vi "Launcher.vi"() -> ()   [LabVIEW 2024]
uses:
  <vilib>/Utility/miscctls.llb/LVRectTypeDef.ctl
  Client/Client_class/Client.lvclass
  5928e640-d91e-4c91-af01-912b1cffb1fd.vi
panel:
  out "Cover Files":path[](array[path])
  in  "Stop":bool
  in  "Hamburger Menu Background":T1
  out "Current Song Name":string
  in  "Stop Button":bool
  in  "Skip Button":bool
  in  "PlayPause Button":bool
  in  "Rewind Button":bool
  out "Music Duration Slider":dbl(slide) scale=0.0..4.590585034013605
  out "Middle Pic":picture
  out "Left Pic":picture
  out "Right Pic":picture
  out "Left Pic 2":picture
  out "Right Pic 2":picture
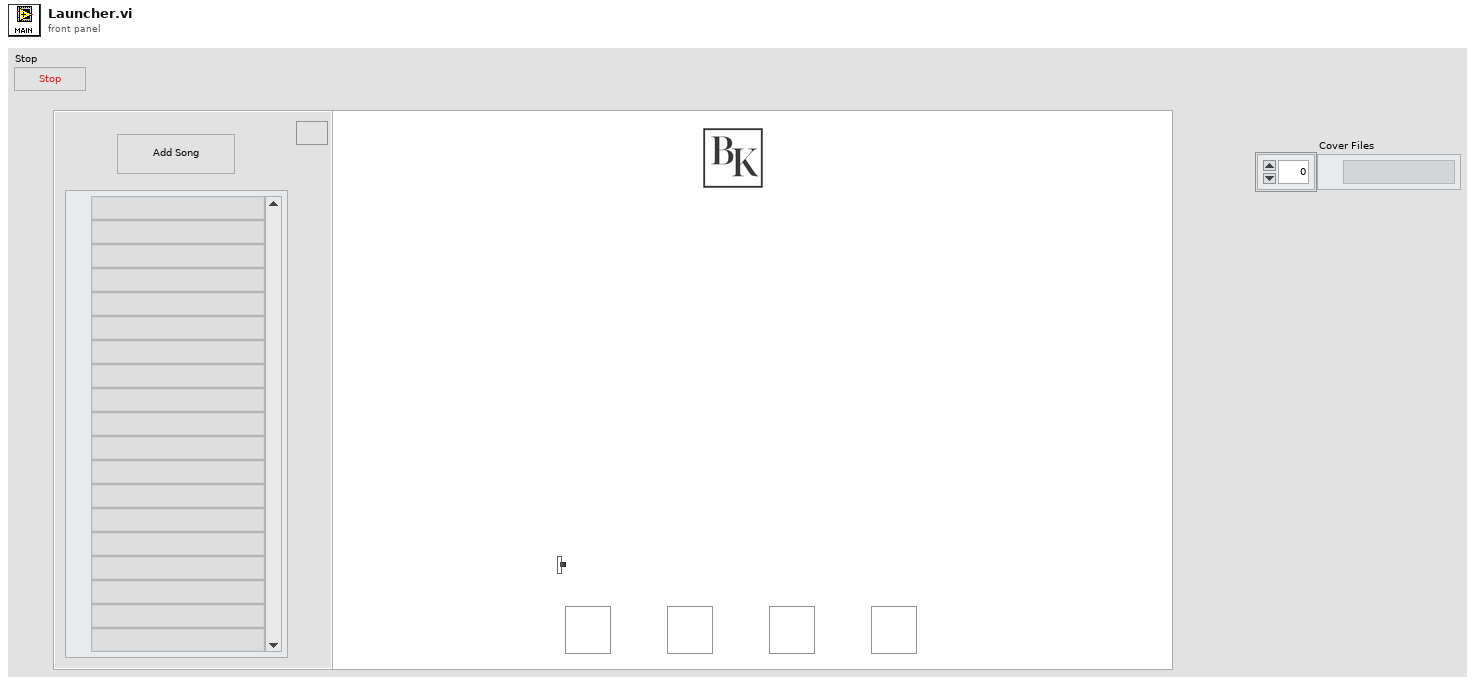
[diagram p1: front panel]
types:
  T1 = cluster{"Hamburger Menu":bool, "New Song":bool, "Song List":path[]}
  T2 = typedef "LVRectTypeDef.ctl" = cluster{"Left":i16, "Top":i16, "Right":i16, "Bottom":i16}
  T3 = cluster{"left":i16, "top":i16, "right":i16, "bottom":i16}
  T4 = typedef "MediaPlayer.lvclass/Current Info.ctl" = cluster{"Duration":dbl, "Name":string, "Is playing?":bool, "Current Music Index":i64}
  T5 = typedef "imagedata.ctl" = cluster{"image type":i32, "image depth":i32, "image":u8[], "mask":u8[], "colors":u32[], "Rectangle":cluster{"left":i16, "top":i16, "right":i16, "bottom":i16}}
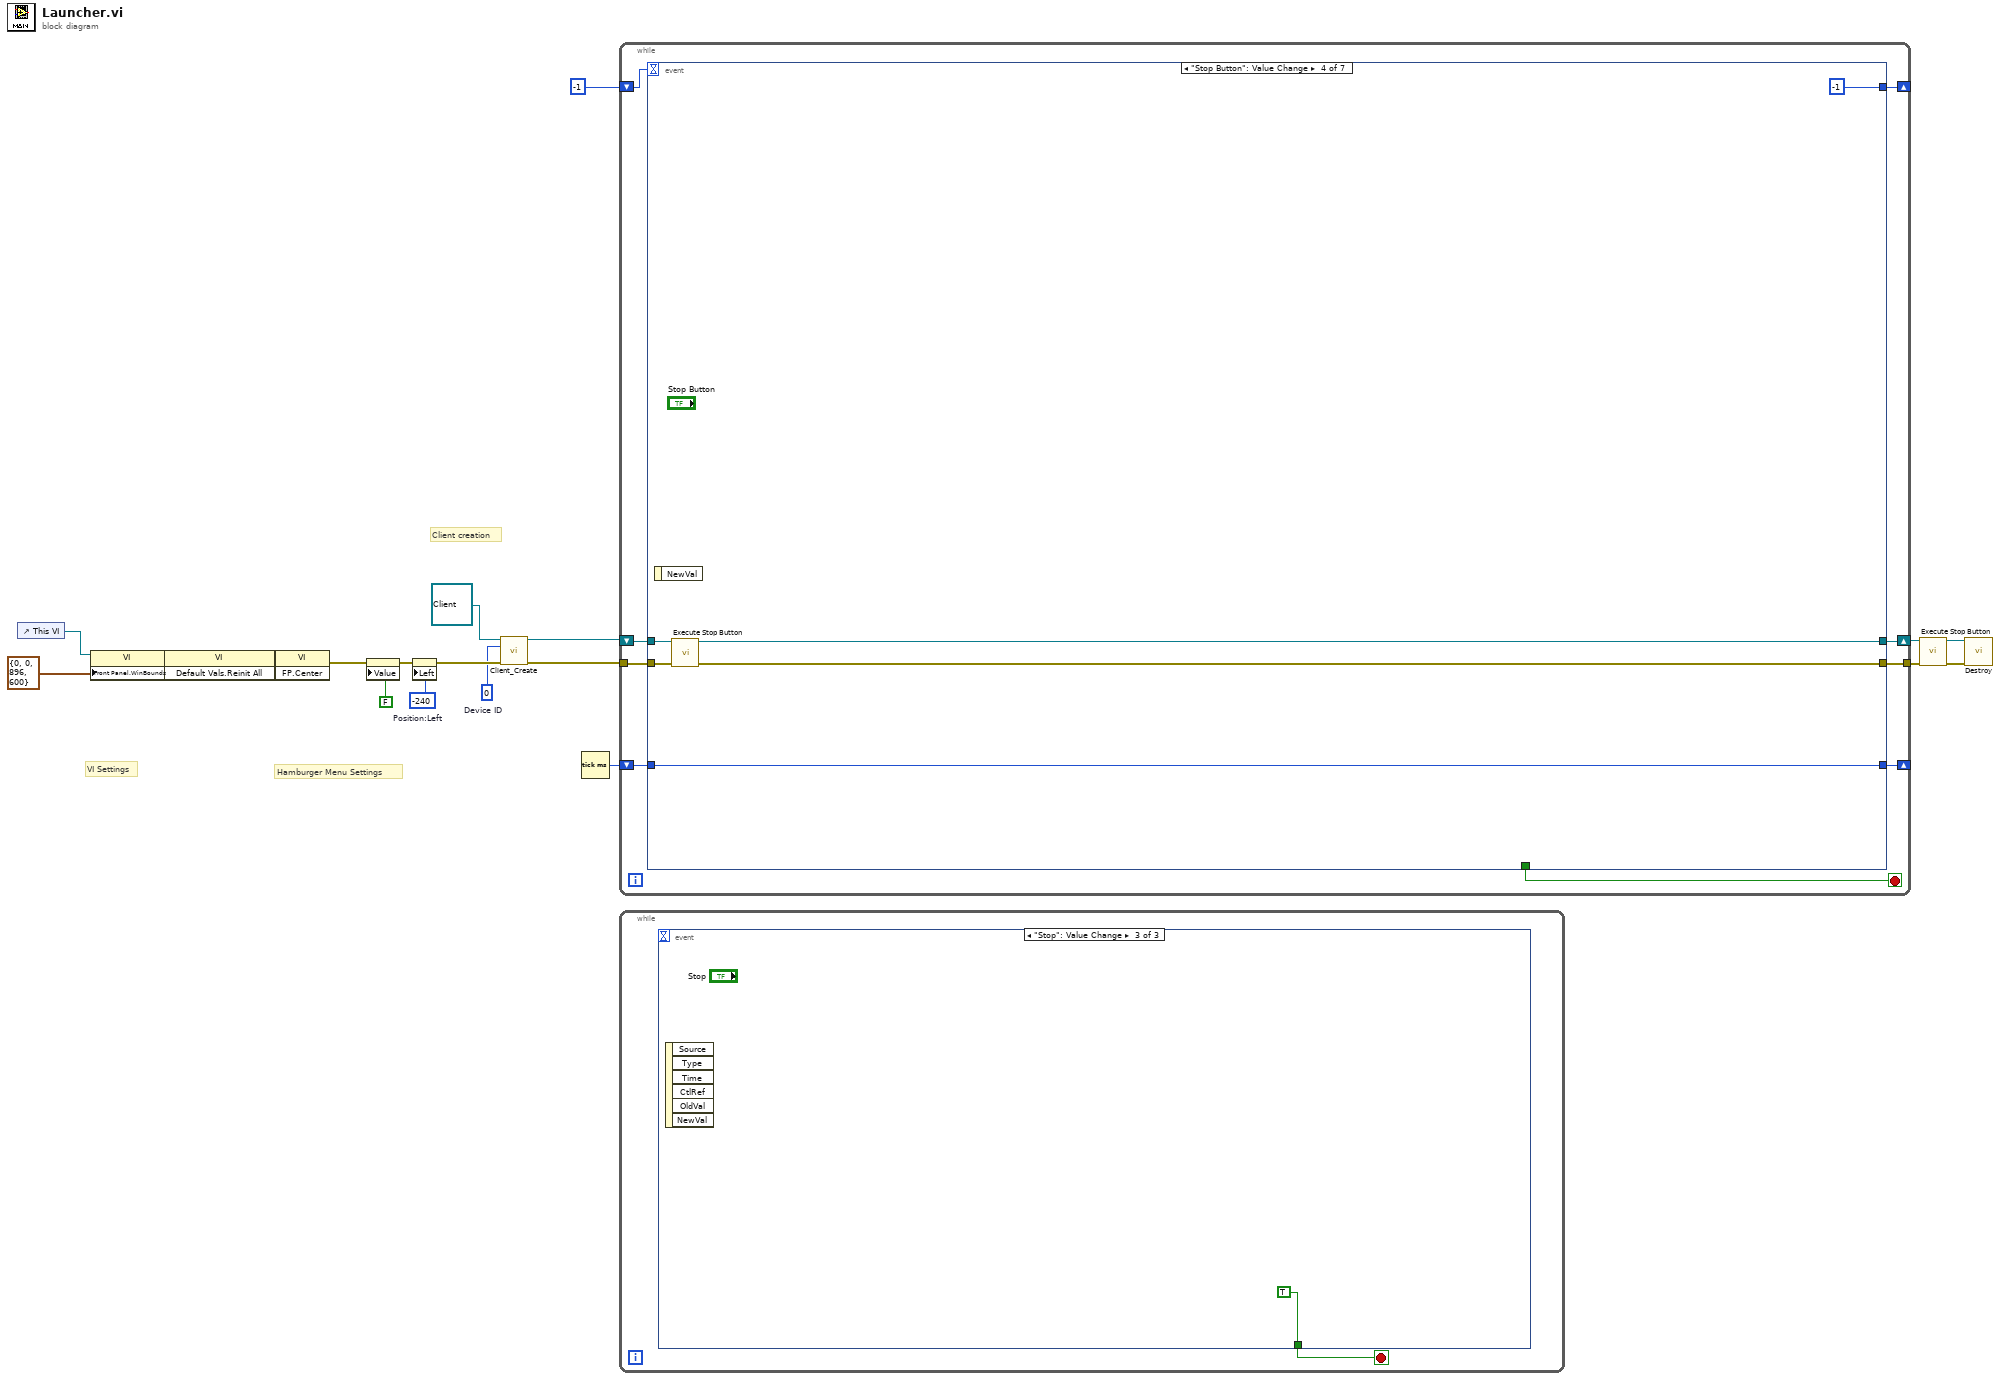
[diagram p0: block diagram]
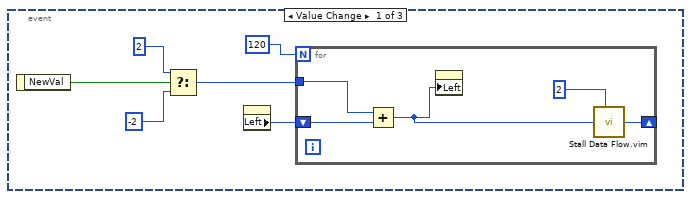
[diagram p2: hidden frame]
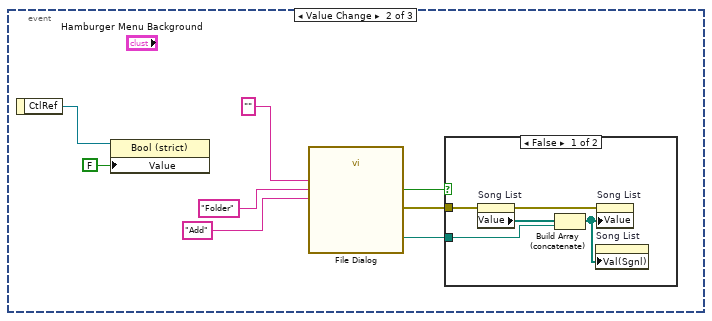
[diagram p3: hidden frame]
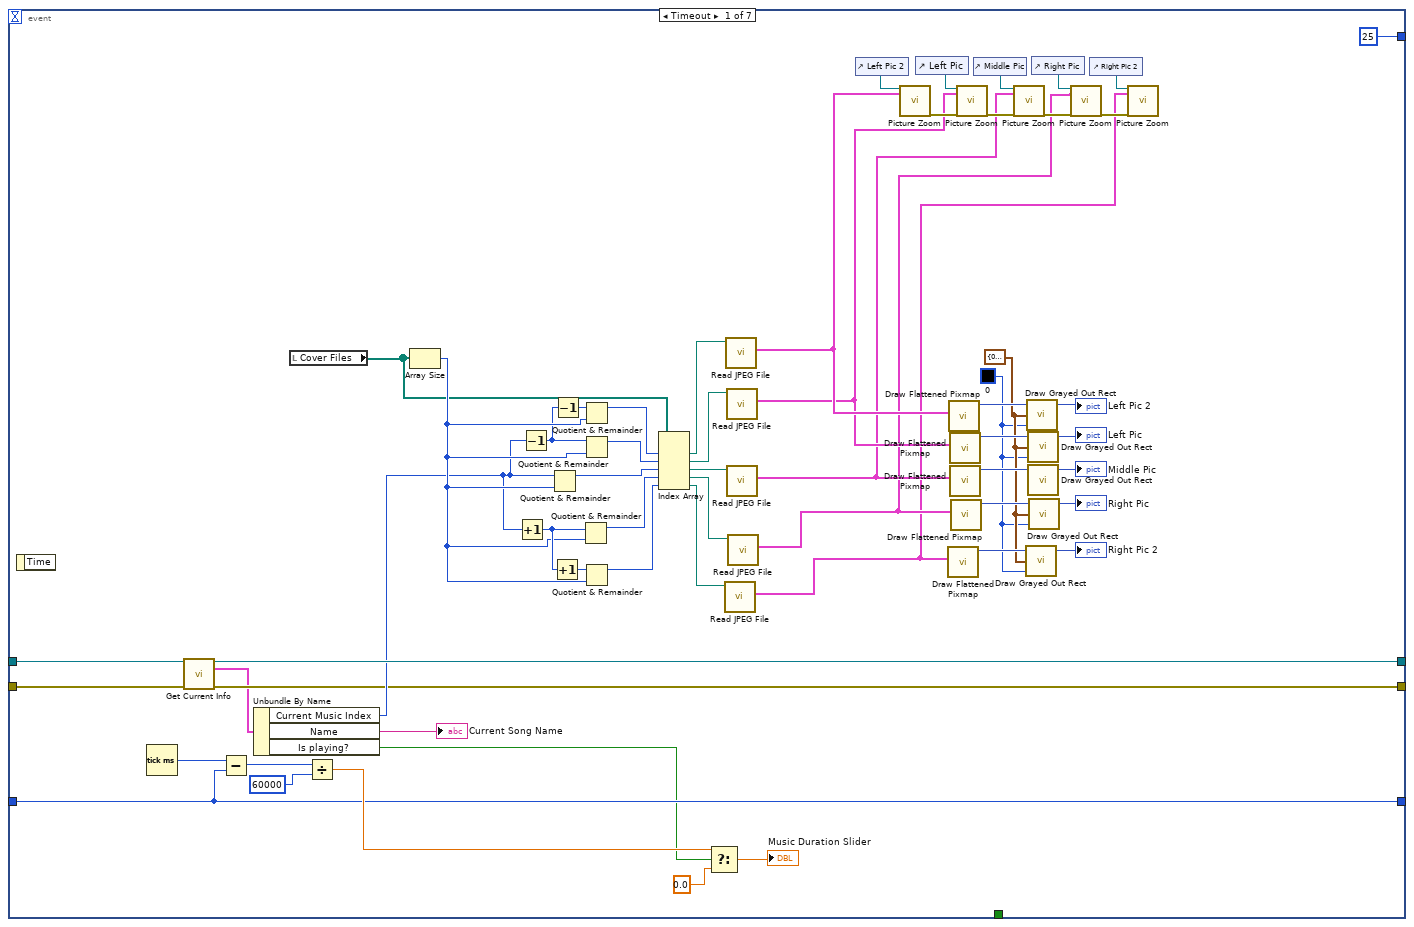
[diagram p5: hidden frame]
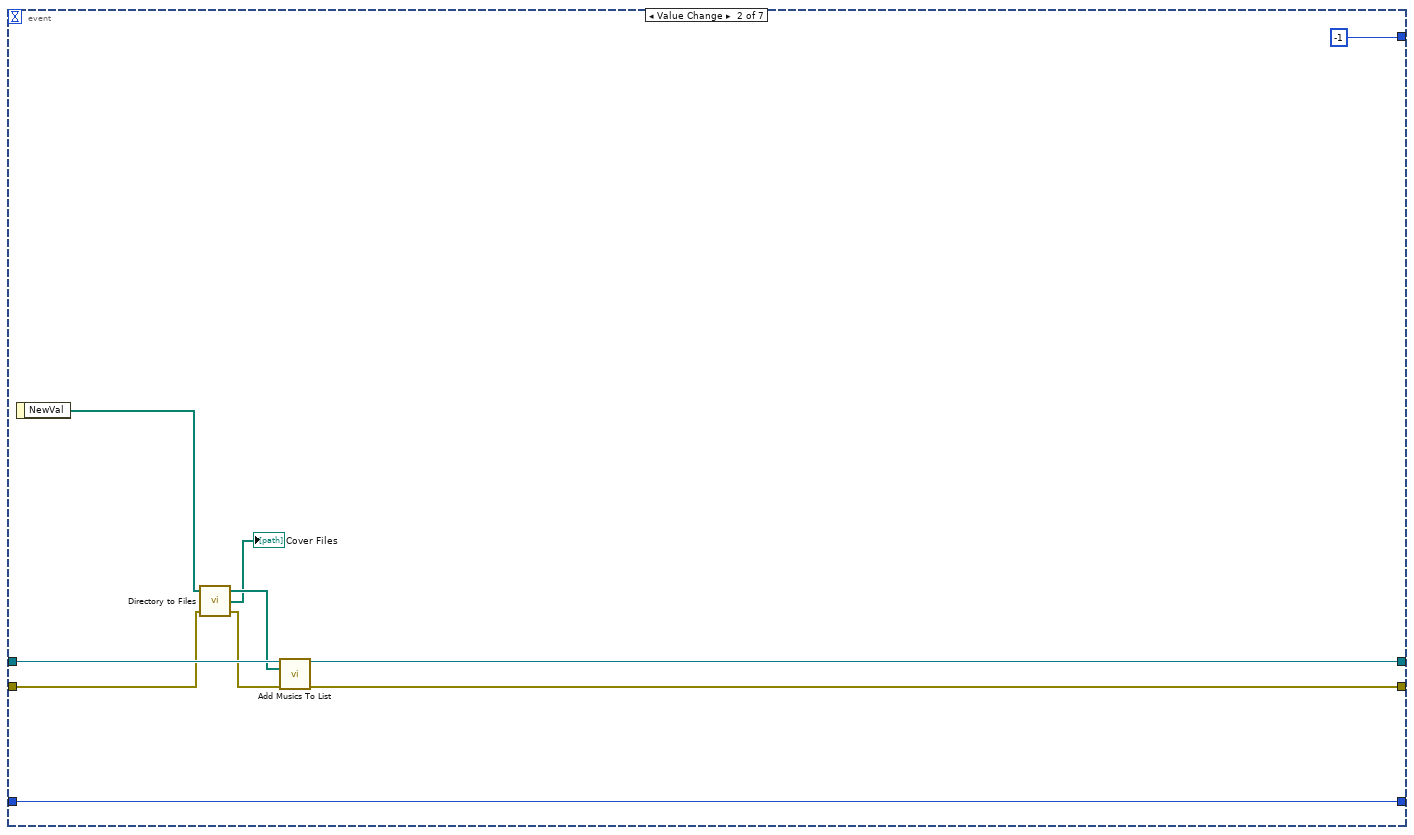
[diagram p6: hidden frame]
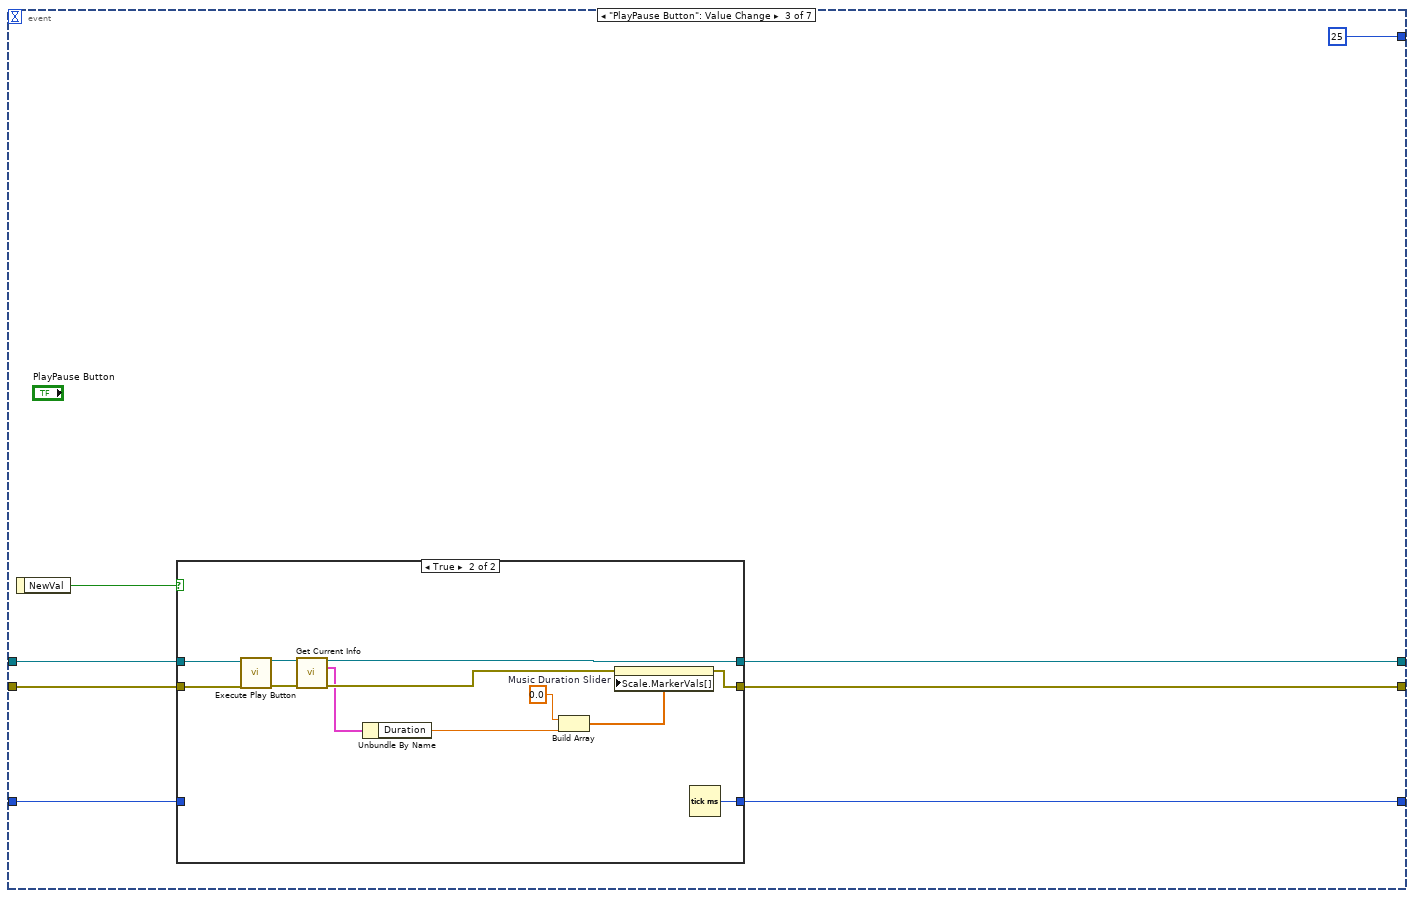
[diagram p7: hidden frame]
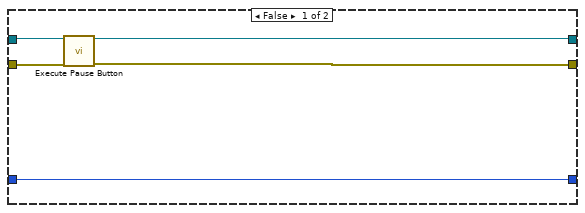
[diagram p8: hidden frame]
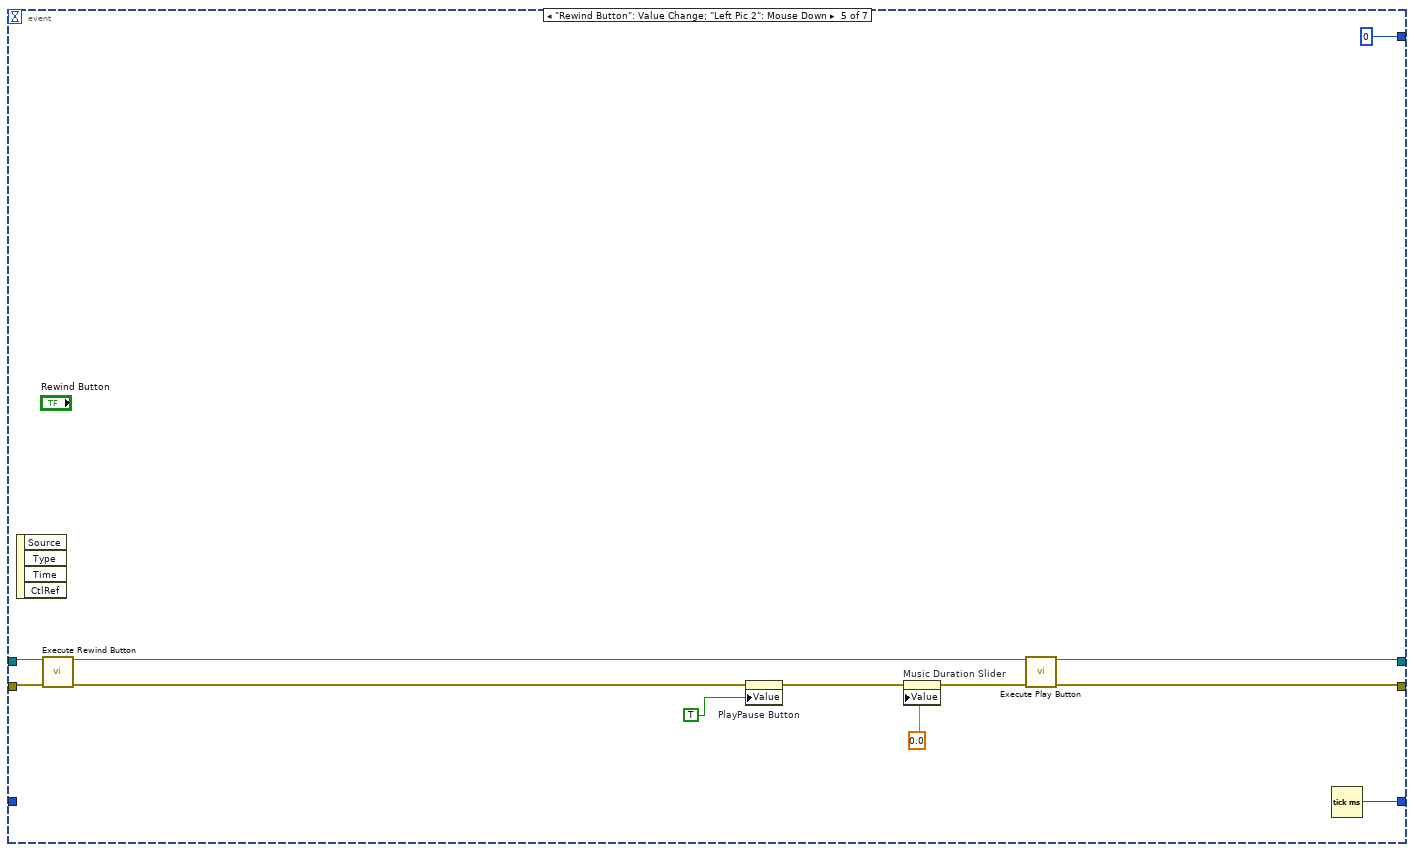
[diagram p9: hidden frame]
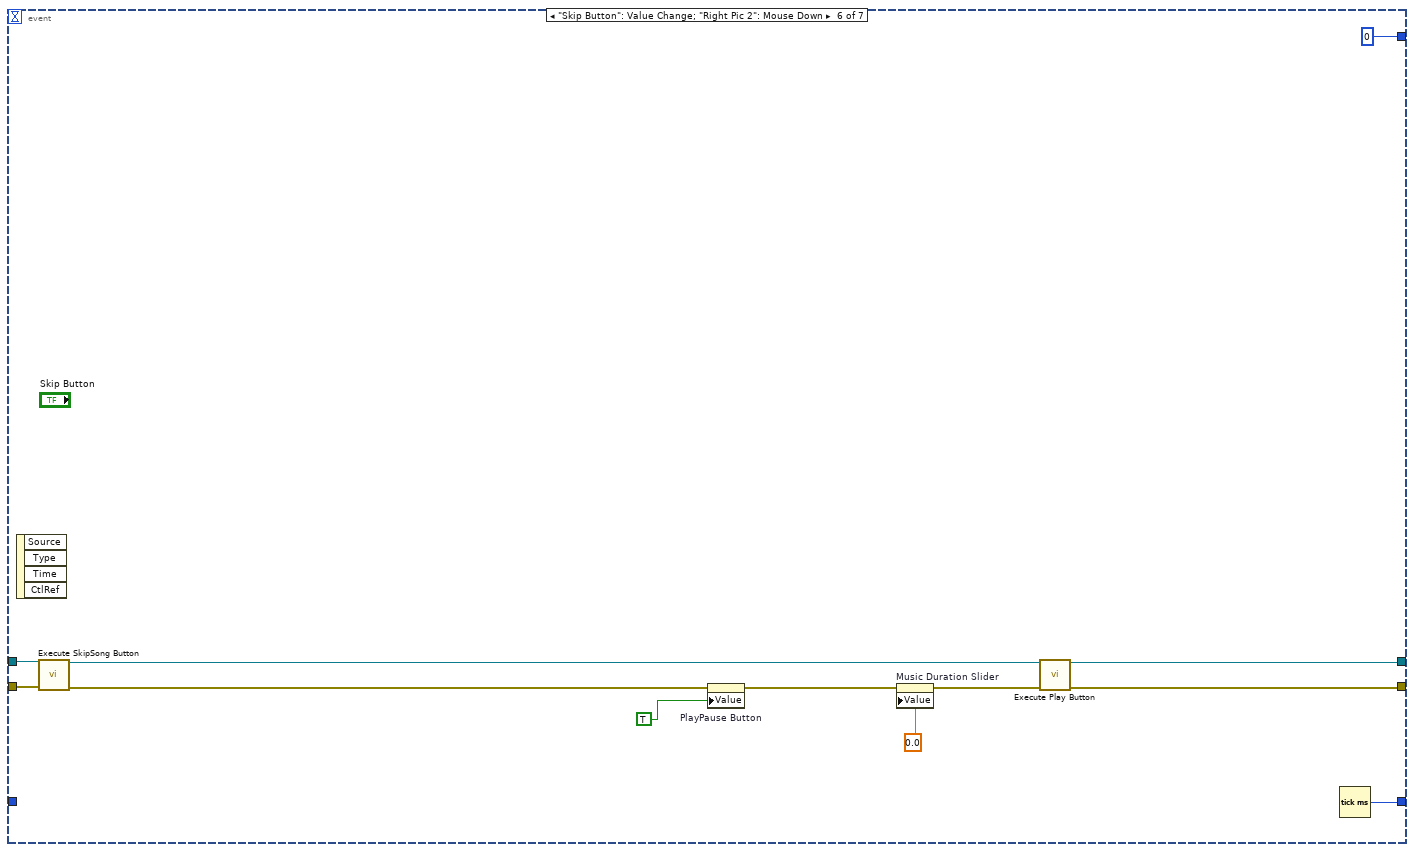
[diagram p10: hidden frame]
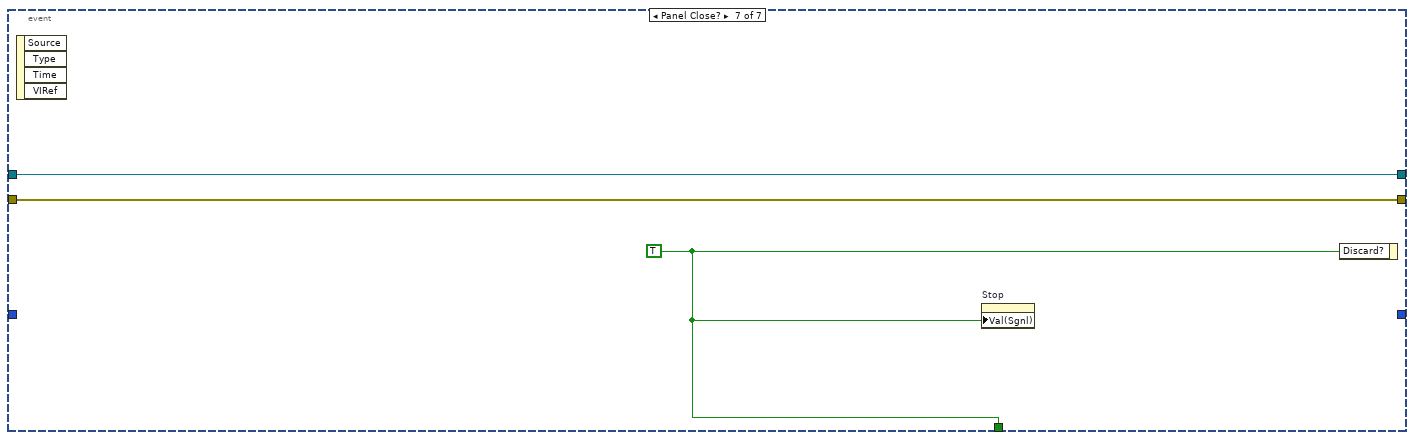
[diagram p11: hidden frame]
diagram:
  w3 = u32 0  # Device ID
  w18 = -240  # Position:Left
  # "Client creation"
  # "VI Settings"
  # "Hamburger Menu Settings"
  n1 = control-ref of="This VI"() -> (w20:refnum<vi>)
  n2 = property class="VI"(reference=w20, "Front Panel.WinBounds"=T2 {"Left"=0, "Top"=0, "Right"=896, "Bottom"=600} ("Front Panel Window:Window Bounds")) -> (reference out=w6:refnum<vi>, error out=w19:errorcluster)  [unwired: 1 in]
  n3 = invoke class="VI" method="Default Vals.Reinit All"(reference=w6, error in=w19) -> (reference out=w5:refnum<vi>, error out=w7:errorcluster)  [unwired: 1 in, 1 out]
  n4 = invoke class="VI" method="FP.Center"(reference=w5, error in=w7) -> (error out=w15:errorcluster)  [unwired: 1 in, 2 out]
  n5 = property on="Hamburger Menu" class="Bool (strict)"(error in=w15, "Value"=FALSE) -> (error out=w17:errorcluster)  [unwired: 1 in, 1 out]
  n6 = property on="Hamburger Menu Background" class="Clust (strict)"(error in=w17, "Left"=w18) -> (error out=w14:errorcluster)  [unwired: 1 in, 1 out]
  n7 = call "Client_Create.vi"("reference in"=refnum<class "Client.lvclass"> refnum ("Client"), "Device ID"=w3, "Error In"=w14) -> ("reference out"=w2:refnum<class "Client.lvclass">, "Error Out"=w1:errorcluster)  [unwired: 11 in]
  n8 = Tick Count (ms)() -> (millisecond timer value=w13:u32)
  n9 = while {
    shift-right: [w27] -> w9
    shift-left: w2 -> [w29]
    tunnel: w1 -> [w28]
    tunnel: [w26] -> w10
    shift-right: [w24] -> _
    shift-left: w13 -> [w25]
    shift-right: [w22] -> _
    shift-left: -1 -> [w23]
    stop <- w30 stop-if-true
    n10 = event shown="[3] \"Stop Button\": Value Change" {
      selector: _ -> [_ _ _ _ _ _ _]
      dyn-events: _ -> [_ _ _ _ _ _ _]
      timeout: w23 -> [_ _ _ _ _ _ _]
      tunnel: [_ _ _ _ _ _ w154] -> w30
      tunnel: w29 -> [w83 w95 w105 w128 w141 w152 w156]
      tunnel: w28 -> [w82 w92 w106 w129 w140 w153 w155]
      tunnel: [w84 w94 w103 w127 w136 w148 w156] -> w27
      tunnel: [w32 w96 w104 w126 w138 w150 w155] -> w26
      tunnel: w25 -> [w81 w97 w100 w125 _ _ _]
      tunnel: [w81 w97 w102 w125 w130 w142 _] -> w24
      tunnel: [25 -1 25 -1 0 0 _] -> w22
      event Timeout {
        w47 = u32 0 ("color(black)")
        w48 = T3 {"left"=0, "top"=0, "right"=1000, "bottom"=1000} ("rect")
        n11 = event-data() -> ()  [unwired: 1 in, 1 out]
        n12 = Tick Count (ms)() -> (millisecond timer value=w88:u32)
        n13 = call-dynamic "Get Current Info.vi"("reference in"=w83, "Error In"=w82) -> ("reference out"=w84:refnum<class "Client.lvclass">, "Current Info"=w31:T4, "Error Out"=w32:errorcluster)  [unwired: 11 in]
        n14 = Subtract(x=w88, y=w81) -> (x-y=w87:u32)
        n15 = Unbundle By Name(w31) -> ("Current Music Index"=w52:i64, "Name"=→"Current Song Name":string, "Is playing?"=w50:bool)
        n16 = local read "Cover Files"() -> (w67:path[])
        n17 = Divide(x=w87, y=u32 60000) -> (x/y=w85:dbl)
        n18 = Array Size(array=w67) -> (size(s)=w71:i32)
        n19 = Increment(x=w52) -> (x+1=w73:i64)
        n20 = Decrement(x=w52) -> (x-1=w70:i64)
        n21 = Quotient & Remainder(x=w52, y=w71) -> (x-y*floor(x/y)=w76:i64)  [unwired: 1 out]
        n22 = Increment(x=w73) -> (x+1=w72:i64)
        n23 = Decrement(x=w70) -> (x-1=w69:i64)
        n24 = Quotient & Remainder(x=w73, y=w71) -> (x-y*floor(x/y)=w77:i64)  [unwired: 1 out]
        n25 = Quotient & Remainder(x=w69, y=w71) -> (x-y*floor(x/y)=w74:i64)  [unwired: 1 out]
        n26 = Quotient & Remainder(x=w70, y=w71) -> (x-y*floor(x/y)=w75:i64)  [unwired: 1 out]
        n27 = Quotient & Remainder(x=w72, y=w71) -> (x-y*floor(x/y)=w78:i64)  [unwired: 1 out]
        n28 = Index Array(array=w67, index #1=w74, index #2=w75, index #3=w76, index #4=w77, index #5=w78) -> (element #1=w68:path, element #2=w58:path, element #3=w59:path, element #4=w60:path, element #5=w61:path)
        n29 = Select(t=w85, s=w50, f=0.0) -> (s? t:f=→"Music Duration Slider":dbl)
        n30 = call <vilib>:"Read JPEG File.vi"("path to JPEG file"=w61) -> ("image data"=w33:T5)  [unwired: 8 in, 2 out]
        n31 = call <vilib>:"Read JPEG File.vi"("path to JPEG file"=w68) -> ("image data"=w46:T5)  [unwired: 8 in, 2 out]
        n32 = call <vilib>:"Read JPEG File.vi"("path to JPEG file"=w58) -> ("image data"=w36:T5)  [unwired: 8 in, 2 out]
        n33 = call <vilib>:"Read JPEG File.vi"("path to JPEG file"=w59) -> ("image data"=w35:T5)  [unwired: 8 in, 2 out]
        n34 = call <vilib>:"Read JPEG File.vi"("path to JPEG file"=w60) -> ("image data"=w34:T5)  [unwired: 8 in, 2 out]
        n35 = control-ref of="Left Pic 2"() -> (w45:refnum<vi>)
        n36 = call "Picture Zoom.vi"("Picture in"=w45, "image data"=w46) -> ("error out"=w44:errorcluster)  [unwired: 17 in]
        n37 = control-ref of="Left Pic"() -> (w40:refnum<vi>)
        n38 = call <vilib>:"Draw Flattened Pixmap.vi"("image data"=w33) -> ("new picture"=w57:picture)  [unwired: 8 in]
        n39 = call <vilib>:"Draw Flattened Pixmap.vi"("image data"=w46) -> ("new picture"=w56:picture)  [unwired: 8 in]
        n40 = call <vilib>:"Draw Flattened Pixmap.vi"("image data"=w36) -> ("new picture"=w55:picture)  [unwired: 8 in]
        n41 = call <vilib>:"Draw Flattened Pixmap.vi"("image data"=w35) -> ("new picture"=w54:picture)  [unwired: 8 in]
        n42 = call <vilib>:"Draw Flattened Pixmap.vi"("image data"=w34) -> ("new picture"=w53:picture)  [unwired: 8 in]
        n43 = call "Picture Zoom.vi"("Picture in"=w40, "image data"=w36, "error in"=w44) -> ("error out"=w43:errorcluster)  [unwired: 16 in]
        n44 = control-ref of="Middle Pic"() -> (w39:refnum<vi>)
        n45 = call "Picture Zoom.vi"("Picture in"=w39, "image data"=w35, "error in"=w43) -> ("error out"=w42:errorcluster)  [unwired: 16 in]
        n46 = call <vilib>:"Draw Grayed Out Rect.vi"("color(black)"=w47, "rect"=w48, "picture"=w57) -> ("new picture"=→"Right Pic 2":picture)  [unwired: 2 in]
        n47 = call <vilib>:"Draw Grayed Out Rect.vi"("color(black)"=w47, "rect"=w48, "picture"=w56) -> ("new picture"=→"Left Pic 2":picture)  [unwired: 2 in]
        n48 = call <vilib>:"Draw Grayed Out Rect.vi"("color(black)"=w47, "rect"=w48, "picture"=w55) -> ("new picture"=→"Left Pic":picture)  [unwired: 2 in]
        n49 = call <vilib>:"Draw Grayed Out Rect.vi"("picture"=w54) -> ("new picture"=→"Middle Pic":picture)  [unwired: 4 in]
        n50 = call <vilib>:"Draw Grayed Out Rect.vi"("color(black)"=w47, "rect"=w48, "picture"=w53) -> ("new picture"=→"Right Pic":picture)  [unwired: 2 in]
        n51 = control-ref of="Right Pic"() -> (w38:refnum<vi>)
        n52 = call "Picture Zoom.vi"("Picture in"=w38, "image data"=w34, "error in"=w42) -> ("error out"=w41:errorcluster)  [unwired: 16 in]
        n53 = control-ref of="Right Pic 2"() -> (w37:refnum<vi>)
        n54 = call "Picture Zoom.vi"("Picture in"=w37, "image data"=w33, "error in"=w41) -> ()  [unwired: 16 in, 1 out]
      }
      event "Hamburger Menu Background.Song List": Value Change {
        n55 = event-data() -> ("NewVal"=w93:path[])  [unwired: 1 in]
        n56 = call "Directory to Files.vi"("error in"=w92, "Directory Path"=w93) -> ("error out"=w91:errorcluster, "Cover Files"=→"Cover Files":path[], "Music Files"=w90:path[])  [unwired: 1 in]
        n57 = call-dynamic "Add Musics To List.vi"("reference in"=w95, "Music List"=w90, "Error In"=w91) -> ("reference out"=w94:refnum<class "Client.lvclass">, "Error Out"=w96:errorcluster)  [unwired: 11 in]
      }
      event "PlayPause Button": Value Change {
        n58 = event-data() -> ("NewVal"=w101:bool)  [unwired: 1 in]
        n59 = case shown="True" w101 {
          tunnel: w106 -> [w108 w120]
          tunnel: w105 -> [w111 w119]
          tunnel: [w109 w117] -> w104
          tunnel: [w110 w113] -> w103
          tunnel: [w107 w118] -> w102
          tunnel: w100 -> [w107 _]
          frame False {
            n60 = call-dynamic "Execute Pause Button.vi"("reference in"=w111, "Error In"=w108) -> ("reference out"=w110:refnum<class "Client.lvclass">, "Error Out"=w109:errorcluster)  [unwired: 12 in]
          }
          frame True {
            n61 = call-dynamic "Execute Play Button.vi"("reference in"=w119, "Error In"=w120) -> ("reference out"=w114:refnum<class "Client.lvclass">, "Error Out"=w116:errorcluster)  [unwired: 12 in]
            n62 = call-dynamic "Get Current Info.vi"("reference in"=w114, "Error In"=w116) -> ("reference out"=w113:refnum<class "Client.lvclass">, "Current Info"=w112:T4, "Error Out"=w115:errorcluster)  [unwired: 11 in]
            n63 = Unbundle By Name(w112) -> ("Duration"=w121:dbl)
            n64 = Build Array(0.0 ("element"), w121) -> (w122:dbl[])
            n65 = property on="Music Duration Slider" class="Slide (strict)"(error in=w115, "Scale.MarkerVals[]"=w122) -> (error out=w117:errorcluster)  [unwired: 1 in, 1 out]
            n66 = Tick Count (ms)() -> (millisecond timer value=w118:u32)
          }
        }
      }
      event "Stop Button": Value Change {
        n67 = event-data() -> ()  [unwired: 1 in, 1 out]
        n68 = call-dynamic "Execute Stop Button.vi"("reference in"=w128, "Error In"=w129) -> ("reference out"=w127:refnum<class "Client.lvclass">, "Error Out"=w126:errorcluster)  [unwired: 12 in]
      }
      event "Rewind Button": Value Change; "Left Pic 2": Mouse Down {
        n69 = event-data() -> ()  [unwired: 1 in, 4 out]
        n70 = call-dynamic "Execute Rewind Button.vi"("reference in"=w141, "Error In"=w140) -> ("reference out"=w137:refnum<class "Client.lvclass">, "Error Out"=w134:errorcluster)  [unwired: 12 in]
        n71 = property on="PlayPause Button" class="Bool (strict)"(error in=w134, "Value"=TRUE ("PlayPause Button")) -> (error out=w133:errorcluster)  [unwired: 1 in, 1 out]
        n72 = property on="Music Duration Slider" class="Slide (strict)"(error in=w133, "Value"=0.0 ("Music Duration Slider")) -> (error out=w132:errorcluster)  [unwired: 1 in, 1 out]
        n73 = call-dynamic "Execute Play Button.vi"("reference in"=w137, "Error In"=w132) -> ("reference out"=w136:refnum<class "Client.lvclass">, "Error Out"=w138:errorcluster)  [unwired: 12 in]
        n74 = Tick Count (ms)() -> (millisecond timer value=w130:u32)
      }
      event "Skip Button": Value Change; "Right Pic 2": Mouse Down {
        n75 = event-data() -> ()  [unwired: 1 in, 4 out]
        n76 = call-dynamic "Execute SkipSong Button.vi"("reference in"=w152, "Error In"=w153) -> ("reference out"=w149:refnum<class "Client.lvclass">, "Error Out"=w147:errorcluster)  [unwired: 12 in]
        n77 = property on="PlayPause Button" class="Bool (strict)"(error in=w147, "Value"=TRUE ("PlayPause Button")) -> (error out=w144:errorcluster)  [unwired: 1 in, 1 out]
        n78 = property on="Music Duration Slider" class="Slide (strict)"(error in=w144, "Value"=0.0 ("Music Duration Slider")) -> (error out=w143:errorcluster)  [unwired: 1 in, 1 out]
        n79 = call-dynamic "Execute Play Button.vi"("reference in"=w149, "Error In"=w143) -> ("reference out"=w148:refnum<class "Client.lvclass">, "Error Out"=w150:errorcluster)  [unwired: 12 in]
        n80 = Tick Count (ms)() -> (millisecond timer value=w142:u32)
      }
      event Panel Close? {
        w154 = TRUE ("Discard?")
        n81 = event-data() -> ()  [unwired: 1 in, 4 out]
        n82 = property on="Stop" class="Bool (strict)"("Val(Sgnl)"=w154) -> ()  [unwired: 2 in, 2 out]
        n83 = event-data("Discard?"=w154) -> ()  [unwired: 1 in, 1 out]
      }
    }
  }
  n84 = while {
    stop <- w157 stop-if-true
    n85 = event shown="[2] \"Stop\": Value Change" {
      selector: _ -> [_ _ _]
      dyn-events: _ -> [_ _ _]
      timeout: _ -> [_ _ _]
      tunnel: [_ _ TRUE] -> w157
      event "Hamburger Menu Background.Hamburger Menu": Value Change {
        n86 = event-data() -> ("NewVal"=w158:bool)  [unwired: 1 in]
        n87 = Select(t=2 ("x"), s=w158, f=-2) -> (s? t:f=w160:i32)
        n88 = property on="Hamburger Menu Background" class="Clust (strict)"() -> ("Left"=w162:i32)  [unwired: 2 in, 2 out]
        n89 = for {
          N: 120 -> [_]
          shift-right: [w166] -> _
          shift-left: w162 -> [w168]
          tunnel: w160 -> [w165]
          n90 = Add(x=w165, y=w168) -> (x+y=w164:i32)
          n91 = property on="Hamburger Menu Background" class="Clust (strict)"("Left"=w164) -> ()  [unwired: 2 in, 2 out]
          n92 = call "Stall Data Flow.vim"("value in"=w164, "milliseconds to wait"=u32 2 ("x+y")) -> ("value out"=w166:i32)  [unwired: 1 out]
        }
      }
      event "Hamburger Menu Background.New Song": Value Change {
        n93 = event-data() -> ("CtlRef"=w170:refnum<vi>)  [unwired: 1 in]
        n94 = property class="Bool (strict)"(reference=w170, "Value"=FALSE) -> ()  [unwired: 1 in, 2 out]
        n95 = call "File Dialog"("button label"="Add", "pattern (all files)"="", "pattern label"="Folder") -> ("selected path"=w172:path, "cancelled"=w171:bool, "error out"=w173:errorcluster)  [unwired: 9 in, 1 out]
        n96 = case shown="False" w171 {
          tunnel: w173 -> [w181 _]
          tunnel: w172 -> [w180 _]
          frame False {
            n97 = property on="Song List" class="Arr (strict)"(error in=w181) -> (error out=w178:errorcluster, "Value"=w179:path[])  [unwired: 1 in, 1 out]
            n98 = Build Array (concatenate)(w179, w180) -> (w177:path[])
            n99 = property on="Song List" class="Arr (strict)"("Val(Sgnl)"=w177) -> ()  [unwired: 2 in, 2 out]
            n100 = property on="Song List" class="Arr (strict)"(error in=w178, "Value"=w177) -> ()  [unwired: 1 in, 2 out]
          }
          frame True {
          }
        }
      }
      event "Stop": Value Change {
        n101 = event-data() -> ()  [unwired: 1 in, 6 out]
      }
    }
  }
  n102 = call-dynamic "Execute Stop Button.vi"("reference in"=w9, "Error In"=w10) -> ("reference out"=w11:refnum<class "Client.lvclass">, "Error Out"=w12:errorcluster)  [unwired: 12 in]
  n103 = call-dynamic "Destroy.vi"("reference in"=w11, "Error In"=w12) -> ()  [unwired: 12 in, 2 out]
